vi "Teleop.vi"(10 "Match Info":T2={"Autonomous Elapsed Seconds"=0.0, "TeleOp Elapsed Seconds"=0.0, "Disabled Elapsed Seconds"=0.0, "Visited Autonomous"=FALSE, "Visited TeleOp"=FALSE, "Visited Disabled"=FALSE, "Autonomous Settings"={"Autonomous Style"=enum."Independent", "VI Refnum"=refnum}}, 11 "Call Context":T3) -> ()   [LabVIEW 2014]
doc: "This VI is called for each TeleOp packet received from the DS where the robot is not disabled. It is often used to read from the joysticks and update I/O or to update setpoints for timed control loops. It should complete and return within 20 milliseconds or it may miss DS packets."
uses:
  <vilib>/Rock Robotics/WPI/DriverStation/WPI_DriverStationDerivedRobotMode.ctl
  <vilib>/Rock Robotics/WPI/DriverStation/WPI_DriverStationMatch Info.ctl
  <vilib>/Rock Robotics/WPI/Joystick/WPI_JoystickGetSetRefNum.vi
  <vilib>/Rock Robotics/Network Tables/SD Write Boolean Array.vi
  <vilib>/Rock Robotics/Network Tables/SD Write Numeric Array.vi
  <vilib>/Rock Robotics/Network Tables/SD Write Boolean.vi
  <vilib>/Rock Robotics/Network Tables/SD Read Boolean.vi
  <vilib>/Rock Robotics/Network Tables/SD Read Number.vi
panel:
  out "Chassis System Reported Status":T1 {"Rotation Status" items=["no Rotation motor output", "Rotate Right", "Rotate Left"]; "X status" items=["no X motor output", "Strafe Right", "Strafe Left"]; "Y status" items=["no Y motor output", "Drive Forward", "Drive Backward"]}
  in  "PID constants":dbl[](array[numeric])
  out "max rate":dbl
  out "Average Distance":dbl
  out "z":dbl
  out "y":dbl
  out "x":dbl
  out "z acceleration":u8(slide) scale=-8.0..8.0
  out "x acceleration":u8(slide) scale=-8.0..8.0
  out "y acceleration":u8(slide) scale=-8.0..8.0
  out "Gyro Angle":dbl
  out "Gyro Angle":dbl(knob) scale=-360.0..360.0
  out "Right Rear Encoder":dbl
  out "Right Front Encoder":dbl
  out "Left Front Encoder":dbl
  out "Left Rear Encoder":dbl
  out "Sample Slider 0":dbl(slide) scale=0.0..5.0
  out "Sample Boolean 1":bool
  out "Sample Boolean 0":bool
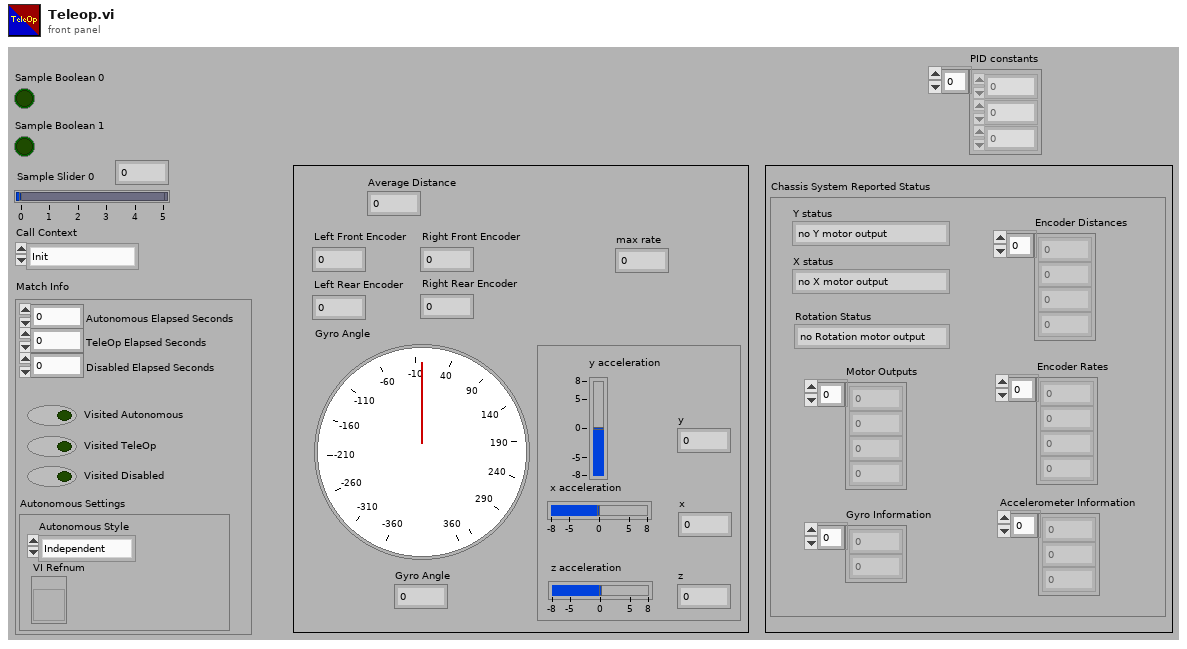
[diagram p1: front panel]
types:
  T1 = cluster{"Y status":u16, "X status":u16, "Rotation Status":u16, "Motor Outputs":dbl[], "Encoder Distances":dbl[], "Encoder Rates":dbl[], "Gyro Information":dbl[], "Accelerometer Information":dbl[]}
  T2 = typedef "WPI_DriverStationMatch Info.ctl" = cluster{"Autonomous Elapsed Seconds":dbl, "TeleOp Elapsed Seconds":dbl, "Disabled Elapsed Seconds":dbl, "Visited Autonomous":bool, "Visited TeleOp":bool, "Visited Disabled":bool, "Autonomous Settings":cluster{"Autonomous Style":enum16{"Iterative", "Independent"}, "VI Refnum":refnum<vi>}}
  T3 = typedef "WPI_DriverStationDerivedRobotMode.ctl" = enum16{"Init", "Execute", "Stop"}
  T4 = typedef "WPI_EncoderDevRef.ctl" = cluster{"DevStatus":errorcluster, "EncoderIndex":T5, "CounterIndex":T6, "DistancePerCount":dbl, "Decoding Type":T7}
  T5 = typedef "FPGA_EncoderIdx.ctl" = enum8{"Enc 0", "Enc 1", "Enc 2", "Enc 3", "Enc 4", "Enc 5", "Enc 6", "Enc 7", "Invalid"}
  T6 = typedef "FPGA_CounterCtrSystemIndex.ctl" = enum8{"Ctr 0", "Ctr 1", "Ctr 2", "Ctr 3", "Ctr 4", "Ctr 5", "Ctr 6", "Ctr 7", "Invalid"}
  T7 = typedef "WPI_EncoderType.ctl" = enum16{"1x", "2x", "4x"}
  T8 = typedef "WPI_GyroDevRef.ctl" = cluster{"DevStatus":errorcluster, "Analog Module":T9, "Analog Channel":T10, "Offset":dbl, "Gain (VoltsPerDegree/Second)":dbl}
  T9 = typedef "FPGA_TypedefAnalogModule.ctl" = enum16{"Controller 1"}
  T10 = typedef "FPGA_AIChannel.ctl" = enum8{"AI 0", "AI 1", "AI 2", "AI 3", "AI MXP 0", "AI MXP 1", "AI MXP 2", "AI MXP 3", "Invalid"}
  T11 = typedef "WPI_AccelerometerDevRef.ctl" = cluster{"DevStatus":errorcluster, "Controller":T9, "Scaling":T12, "Analog Channels":T13, "I2C Bus":T14, "SPI Bus":T15, "Accel Range":T16, "ADXL345 Axes":T17, "Handle":i32, "Device Address":u8, "Accel Type":enum16{"Analog", "ADXL345 I2C", "ADXL345 SPI", "Internal"}}
  T12 = typedef "WPI_AccelerometerScaling.ctl" = cluster{"Gain (VoltsPerG)":dbl, "Center Voltage":dbl}
  T13 = typedef "WPI_AccelerometerAnalogChannels.ctl" = cluster{"X-Axis":T10, "Y-Axis":T10, "Z-Axis":T10}
  T14 = typedef "i2c_bus.ctl" = enum16{"I2C On-Board", "I2C MXP", "Invalid"}
  T15 = typedef "spi_bus.ctl" = enum16{"SPI On-Board, CS0", "SPI On-Board, CS1", "SPI On-Board, CS2", "SPI On-Board, CS3", "SPI MXP", "Invalid"}
  T16 = typedef "ADXL345 Range.ctl" = u8
  T17 = typedef "WPI_AccelerometerADXL345 Axes.ctl" = cluster{"X-Axis":bool, "Y-Axis":bool, "Z-Axis":bool}
  T18 = cluster{"X-Axis":dbl, "Y-Axis":dbl, "Z-Axis":dbl}
  T19 = typedef "WPI_JoystickDevRef.ctl" = cluster{"Device":T20}
  T20 = typedef "WPI_JoystickDeviceEnum.ctl" = enum16{"USB 0", "USB 1", "USB 2", "USB 3", "USB 4", "USB 5"}
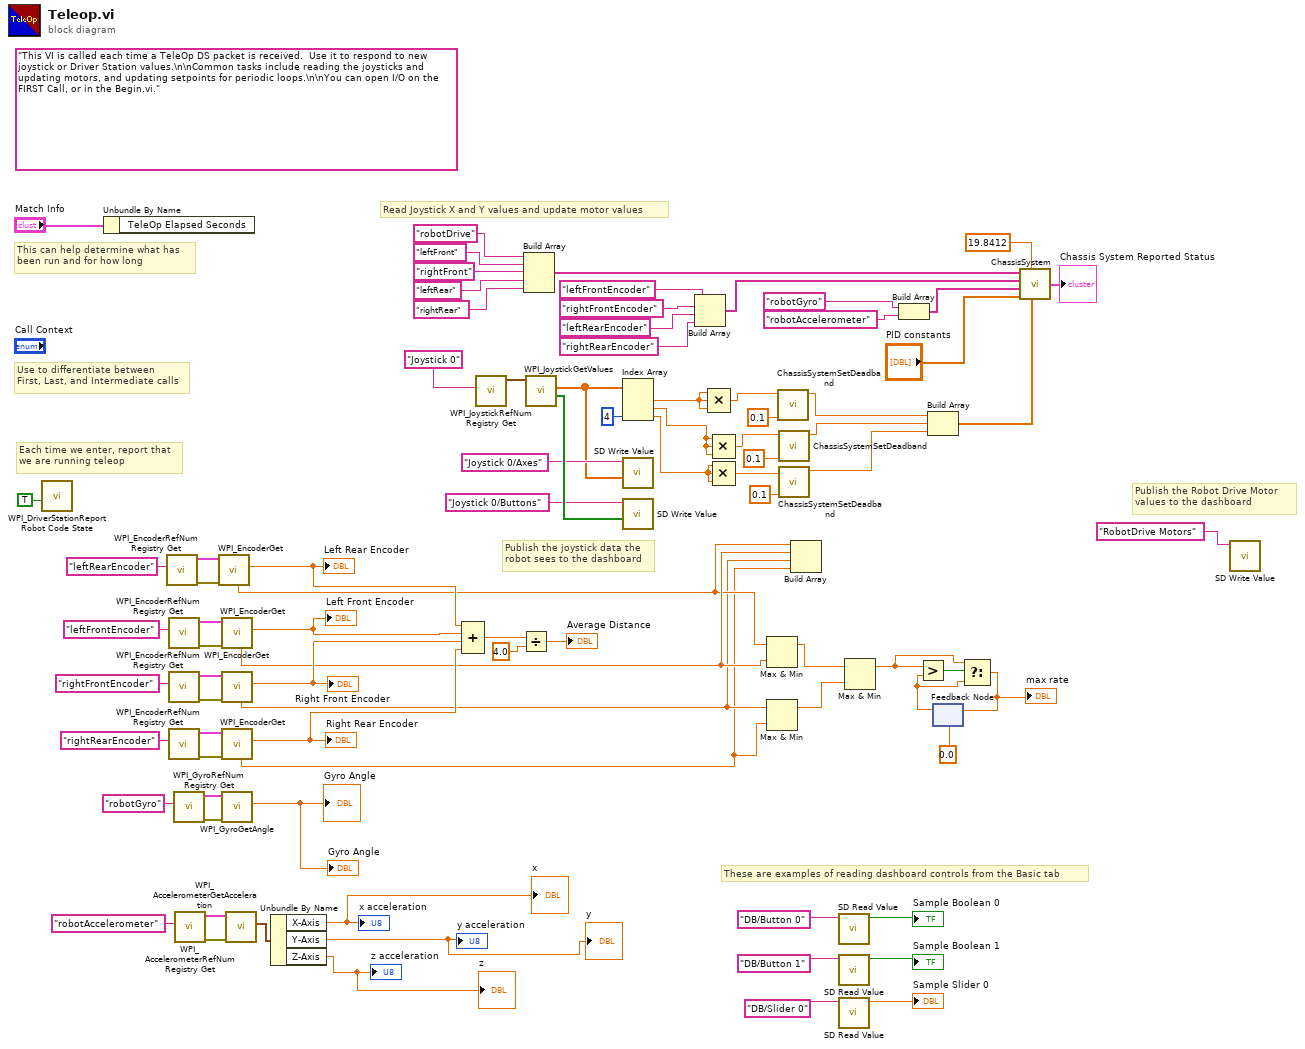
[diagram p0: block diagram]
diagram:
  (unwired) "This VI is called each time a TeleOp DS packet is received.  Use it to respond to new joystick or Driver Station values.\n\nCommon tasks include reading the joysticks and updating motors, and updating setpoints for periodic loops.\n\nYou can open I/O on the FIRST Call, or in the Begin.vi."
  # "These are examples of reading dashboard controls from the Basic tab"
  # "Publish the Robot Drive Motor\nvalues to the dashboard"
  # "Publish the joystick data the\nrobot sees to the dashboard"
  # "Each time we enter, report that\nwe are running teleop"
  # "Use to differentiate between\nFirst, Last, and Intermediate calls"
  # "This can help determine what has\nbeen run and for how long"
  # "Read Joystick X and Y values and update motor values"
  n1 = call <vilib>:"WPI_DriverStationReport Robot Code State.vi"("TeleOp"=TRUE ("Autonomous")) -> ()  [unwired: 10 in, 1 out]
  n2 = Unbundle By Name("Match Info") -> ()  [unwired: 1 out]
  n3 = call <vilib>:"WPI_EncoderRefNum Registry Get.vi"("refnum name"="leftRearEncoder") -> ("error out"=w68:errorcluster, "EncoderDevRef"=w67:T4)  [unwired: 9 in]
  n4 = call <vilib>:"WPI_EncoderRefNum Registry Get.vi"("refnum name"="leftFrontEncoder") -> ("error out"=w65:errorcluster, "EncoderDevRef"=w64:T4)  [unwired: 9 in]
  n5 = call <vilib>:"WPI_EncoderRefNum Registry Get.vi"("refnum name"="rightFrontEncoder") -> ("error out"=w62:errorcluster, "EncoderDevRef"=w61:T4)  [unwired: 9 in]
  n6 = call <vilib>:"WPI_EncoderRefNum Registry Get.vi"("refnum name"="rightRearEncoder") -> ("error out"=w59:errorcluster, "EncoderDevRef"=w58:T4)  [unwired: 9 in]
  n7 = call <vilib>:"WPI_GyroRefNum Registry Get.vi"("refnum name"="robotGyro") -> ("error out"=w50:errorcluster, "GyroDevRef"=w49:T8)  [unwired: 9 in]
  n8 = call <vilib>:"WPI_AccelerometerRefNum Registry Get.vi"("refnum name"="robotAccelerometer") -> ("error out"=w46:errorcluster, "AccelerometerDevRef"=w45:T11)  [unwired: 9 in]
  n9 = call <vilib>:"WPI_EncoderGet.vi"("error in (no error)"=w68, "EncoderDevRef"=w67) -> ("Distance"=w36:dbl, "Rate"=w24:dbl)  [unwired: 4 in, 4 out]
  "Left Rear Encoder" <- w36
  n10 = call <vilib>:"WPI_EncoderGet.vi"("error in (no error)"=w65, "EncoderDevRef"=w64) -> ("Distance"=w35:dbl, "Rate"=w25:dbl)  [unwired: 4 in, 4 out]
  "Left Front Encoder" <- w35
  n11 = call <vilib>:"WPI_EncoderGet.vi"("error in (no error)"=w62, "EncoderDevRef"=w61) -> ("Distance"=w34:dbl, "Rate"=w23:dbl)  [unwired: 4 in, 4 out]
  "Right Front Encoder" <- w34
  n12 = call <vilib>:"WPI_EncoderGet.vi"("error in (no error)"=w59, "EncoderDevRef"=w58) -> ("Distance"=w33:dbl, "Rate"=w22:dbl)  [unwired: 4 in, 4 out]
  "Right Rear Encoder" <- w33
  n13 = call <vilib>:"WPI_GyroGetAngle.vi"("error in (no error)"=w50, "GyroDevRef"=w49) -> ("Angle"=→"Gyro Angle" →"Gyro Angle":dbl)  [unwired: 6 in, 3 out]
  n14 = call <vilib>:"WPI_AccelerometerGetAcceleration.vi"("error in"=w46, "AccelerometerDevRef"=w45) -> ("Accelerations"=w43:T18)  [unwired: 7 in, 2 out]
  n15 = Unbundle By Name(w43) -> ("X-Axis"=→"x acceleration" →"x":dbl, "Y-Axis"=→"y acceleration" →"y":dbl, "Z-Axis"=→"z acceleration" →"z":dbl)
  n16 = Compound Arithmetic op=ADD(w36, w35, w34, w33) -> (w39:dbl)
  n17 = call <vilib>:"WPI_JoystickRefNum Registry Get.vi"("refnum name"="Joystick 0") -> ("JoystickDevRef"=w85:T19)  [unwired: 1 in, 9 out]
  n18 = Divide(x=w39, y=4.0) -> (x/y=→"Average Distance":dbl)
  n19 = Build Array("robotDrive" ("refnum name"), "leftFront", "rightFront" ("refnum name"), "leftRear", "rightRear") -> (w16:string[])
  n20 = call <vilib>:"WPI_JoystickGetValues.vi"("JoystickDevRef"=w85) -> ("Buttons"=w83:bool[], "Axes"=w73:dbl[])  [unwired: 6 in, 3 out]
  n21 = Index Array(array=w73, index #3=4 ("index")) -> (element #1=w69:dbl, element #2=w70:dbl, element #3=w71:dbl)  [unwired: 2 in]
  n22 = call-poly <vilib>:"SD Write Value.vi"("Numeric Array"=w73, "Name"="Joystick 0/Axes") -> ()  [unwired: 8 in, 2 out]
  n23 = call-poly <vilib>:"SD Write Value.vi"("Boolean Array"=w83, "Name"="Joystick 0/Buttons") -> ()  [unwired: 8 in, 2 out]
  n24 = Build Array("leftFrontEncoder", "rightFrontEncoder", "leftRearEncoder", "rightRearEncoder") -> (w11:string[])
  n25 = Compound Arithmetic op=MULTIPLY(w69, w69, w69) -> (w52:dbl)
  n26 = Compound Arithmetic op=MULTIPLY(w70, w70, w70) -> (w54:dbl)
  n27 = Compound Arithmetic op=MULTIPLY(w71, w71, w71) -> (w56:dbl)
  n28 = Max & Min(x=w24, y=w25) -> (max(x,y)=w32:dbl)  [unwired: 1 out]
  n29 = Max & Min(x=w23, y=w22) -> (max(x,y)=w31:dbl)  [unwired: 1 out]
  n30 = call "ChassisSystemSetDeadband.vi"("Deadband"=0.1, "Joystick Axis Value"=w52) -> ("Output Motor Value"=w6:dbl)  [unwired: 9 in]
  n31 = call "ChassisSystemSetDeadband.vi"("Deadband"=0.1, "Joystick Axis Value"=w54) -> ("Output Motor Value"=w5:dbl)  [unwired: 9 in]
  n32 = call "ChassisSystemSetDeadband.vi"("Deadband"=0.1, "Joystick Axis Value"=w56) -> ("Output Motor Value"=w4:dbl)  [unwired: 9 in]
  n33 = Build Array(w24, w25, w23, w22) -> ()  [unwired: 1 out]
  n34 = call-poly <vilib>:"SD Read Value.vi"("Name"="DB/Button 0" ("refnum name")) -> ("Boolean"=→"Sample Boolean 0":bool)  [unwired: 8 in, 2 out]
  n35 = call-poly <vilib>:"SD Read Value.vi"("Name"="DB/Button 1" ("refnum name")) -> ("Boolean"=→"Sample Boolean 1":bool)  [unwired: 8 in, 2 out]
  n36 = call-poly <vilib>:"SD Read Value.vi"("Name"="DB/Slider 0" ("refnum name")) -> ("Numeric"=→"Sample Slider 0":dbl)  [unwired: 8 in, 2 out]
  n37 = Max & Min(x=w32, y=w31) -> (max(x,y)=w28:dbl)  [unwired: 1 out]
  n38 = Build Array("robotGyro", "robotAccelerometer") -> (w8:string[])
  n39 = Build Array(w6, w5, w4) -> (w3:dbl[])
  n40 = feedback #1(0.0) -> (w27:dbl)
  n41 = Greater?(x=w28, y=w27) -> (0:w29:bool)
  n42 = Select(t=w28, s=w29, f=w27) -> (s? t:f=w26:dbl)
  "max rate" <- w26
  n43 = feedback-in #1(w26) -> ()
  n44 = call "ChassisSystem.vi"("Targets"=w3, "Robot Maximum Rate"=19.8412, "PID constants"="PID constants", "Gyro and Accelerometer reference names"=w8, "Encoder Reference names"=w11, "Motor and PWM reference names"=w16) -> ("Reported Status"=→"Chassis System Reported Status":T1)
  n45 = call-poly <vilib>:"SD Write Value.vi"("Name"="RobotDrive Motors") -> ()  [unwired: 9 in, 2 out]
